vi "UTIL Piezo Feat_NoNotch.vi"(7 "Piezo In":waveform(dbl)) -> (1 "Piezo Power":dbl format="%0.2f", 3 "Filtered Piezo Out":waveform(dbl))   [LabVIEW 2010]
doc: "This VI computed the r.m.s. power in the Piezo signal to serve as a surrogate fo EMG power in the task of sleep wake differentiation.\n\nInputs\n Piezo In Waveform\nOutputs\n Piezo Power DBL"
uses:
  <vilib>/Analysis/NI_AALBase.lvlib
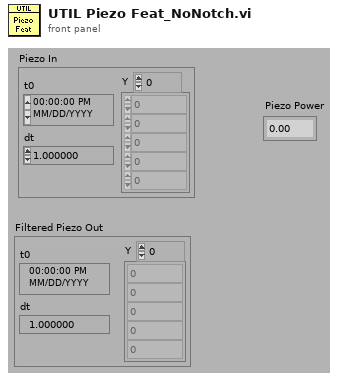
[diagram p1: front panel]
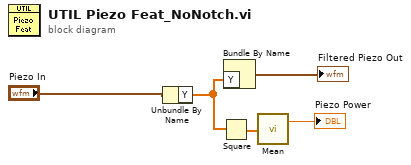
[diagram p0: block diagram]
diagram:
  n1 = Unbundle By Name("Piezo In") -> ("Y"=w1:dbl[])
  n2 = Square(x=w1) -> (x^2=w5:dbl[])
  n3 = Bundle By Name("Y"=w1) -> (→"Filtered Piezo Out":waveform(dbl))  [unwired: 1 in]
  n4 = call <vilib>:"Mean.vi"("X"=w5) -> ("mean"=→"Piezo Power":dbl)  [unwired: 1 out]
